vi "Add Child Tag XML.vi"(4 "Values":string[](array[string]), 6 "Names":string[](array[string]), 8 "Error In":errorcluster, 9 "Tag Name":string, 10 "Parent Node":refnum<k20>, 11 "DOM In":refnum<k20>) -> (0 "Error Out":errorcluster, 1 "Child Node":refnum<k20>, 2 "Parent Node":refnum<k20>, 3 "DOM Out":refnum<k20>)   [LabVIEW 2016, in "Tree Manager.lvclass"]
uses:
  Tree Manager.lvclass
  <resource>/objmgr/DOMUserDefRef.rc
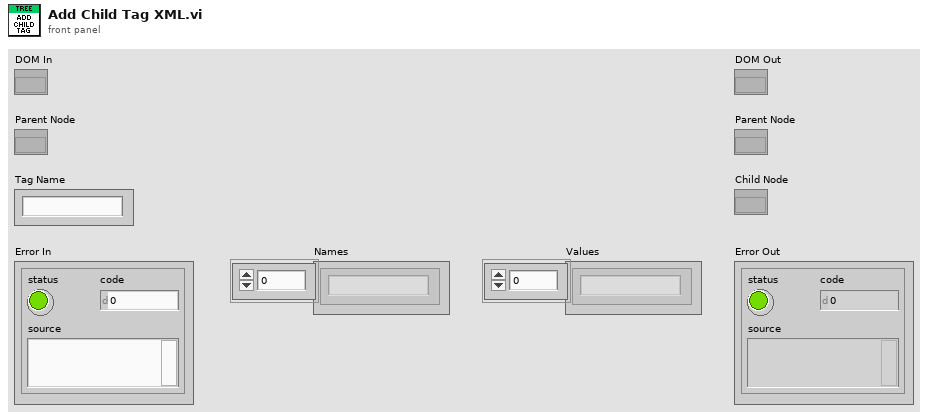
[diagram p1: front panel]
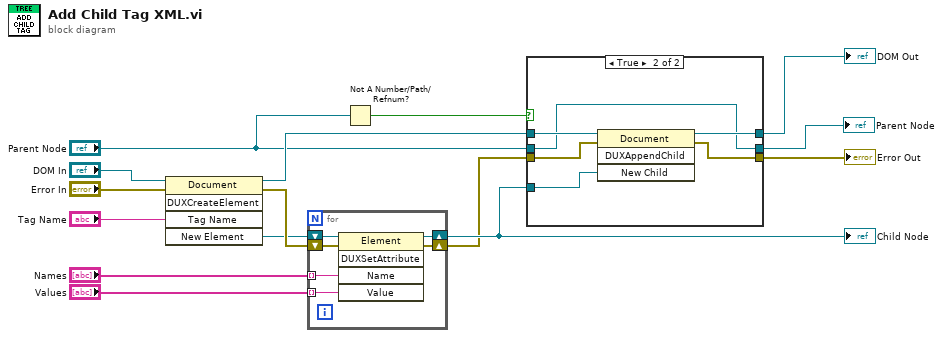
[diagram p0: block diagram]
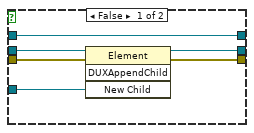
[diagram p2: hidden frame]
diagram:
  n1 = invoke class="Document" method="DUXCreateElement"(reference="DOM In", error in="Error In", "Tag Name"="Tag Name") -> (reference out=w4:refnum<k20>, error out=w12:errorcluster, "New Element"=w9:refnum<k20>)  [unwired: 2 in, 2 out]
  n2 = for {
    tunnel: "Names" -> [w20] mode=indexing
    tunnel: "Values" -> [w19] mode=indexing
    shift-right: [w18] -> w15
    shift-left: w9 -> [w21]
    shift-right: [w16] -> w13
    shift-left: w12 -> [w17]
    n3 = invoke class="Element" method="DUXSetAttribute"(reference=w21, error in=w17, "Name"=w20, "Value"=w19) -> (reference out=w18:refnum<k20>, error out=w16:errorcluster)  [unwired: 1 in, 3 out]
  }
  "Child Node" <- w15
  n4 = Not A Number/Path/Refnum?(number/path/refnum="Parent Node") -> (NaN/Path/Refnum?=w1:bool)
  n5 = case shown="True" w1 {
    tunnel: w15 -> [w27 w31]
    tunnel: w13 -> [w26 w32]
    tunnel: "Parent Node" -> [w25 w28]
    tunnel: [w24 w30] -> w6
    tunnel: [w23 w28] -> w5
    tunnel: w4 -> [w22 w33]
    tunnel: [w22 w29] -> w3
    frame False {
      n6 = invoke class="Element" method="DUXAppendChild"(reference=w25, error in=w26, "New Child"=w27) -> (reference out=w23:refnum<k20>, error out=w24:errorcluster)  [unwired: 1 in, 2 out]
    }
    frame True {
      n7 = invoke class="Document" method="DUXAppendChild"(reference=w33, error in=w32, "New Child"=w31) -> (reference out=w29:refnum<k20>, error out=w30:errorcluster)  [unwired: 1 in, 2 out]
    }
  }
  "Error Out" <- w6
  "DOM Out" <- w3
  "Parent Node" <- w5
